vi "LIA Debugging Host.vi"() -> ()   [LabVIEW 2018]
uses:
  Shared/lib/host/Public/pll settings.ctl
  Shared/lib/host/Public/lock-in settings.ctl
  Class/LIA Debugging.lvclass
  C:/Users/jfernand/Repositories/Lock-In-Amplifier/Shared/lib/interface/Interface/LIA Host Interface.lvclass
  C:/Users/jfernand/Repositories/Lock-In-Amplifier/Shared/lib/interface/Interface FPGA/LIA Host Interface FPGA.lvclass
  <vilib>/Analysis/4window.llb/windowTd.ctl
  <vilib>/measure/maspectr.llb/FFT Power Spectrum and PSD for N Chan.vi
  <vilib>/Utility/error.llb/Error Cluster From Error Code.vi
  <vilib>/rvi/errors/niLvFpgaAdjustHostInterfaceError.vi
  <vilib>/rvi/interface/nirviReadWriteControl/nirviReadWriteControl.xnode
  Shared/lib/host/Lock-In Amplifier Example Host.lvlib
  <vilib>/Analysis/NI_AALPro.lvlib
  <vilib>/measure/NI_MAPro.lvlib
  <vilib>/Analysis/NI_AALBase.lvlib
  NiFpgaLv.dll
  <vilib>/rvi/interface/Simulation/niFpgaSimulationCallBeginRW.vi
  Shared/lib/interface/Interface FPGA/LIA Host Interface FPGA.lvclass
panel:
  in  "Tab Control 2":enum32{"Page 1", "Page 2"}(tab)
  in  "dpll.m 0":i8=-20
  in  "lock-in.decimator0 0":enum16{"None", "CIC", "FIR", "4HB", "SOS"}(ring)=enum."FIR"
  in  "lock-in.decimator1 0":enum16{"None", "FIR", "SOS"}(ring)=enum."FIR"
  in  "lock-in.iir config":T1={"b0"=0.001556396484375, "b1"=-0.000762939453125, "-a1"=1.9305267333984375, "-a2"=-0.9328765869140625} {"b0" format="%.17g"; "b1" format="%.17g"; "-a1" format="%.17g"; "-a2" format="%.17g"}
  out "lock-in.max-min":dbl=1.9775797561733533e-07 caption="Deviation" format="%#_6p"
  out "lock-in.min":dbl=1.9775797561733533e-07 caption="Deviation" format="%#_6p"
  out "lock-in.max":dbl=1.9775797561733533e-07 caption="Deviation" format="%#_6p"
  in  "Tab Control 1":T2(tab)
  out "pll.vco output 0":fxp<+/-,48,0> format="%#.18g"
  out "lock-in.cic config 0":cluster{"factor":fxp<+,16,16>, "shift":i16}
  out "dpll.vco output 0":fxp<+/-,48,0> format="%#.18g"
  out "dpll.config 0":T3
  out "nco.frequency 0":fxp<+/-,48,0>=0.0010000000000012221 format="%#_19g"
  out "stream.state 0":T4(ring)
  out "lock-in.decimator0 0 read":enum16{"None", "CIC", "FIR", "4HB", "SOS"}(ring)
  out "size(s)":i32
  out "lock-in.carrier 0 read":fxp<+/-,48,0> format="%_19g"
  out "stream.overflow? 0":bool
  out "Power Spectrum (dBm)":cluster{"f0":dbl, "df":dbl, "magnitude":dbl[]}(graph)
  out "Waveform Graph 3":dbl[][](graph)
  out "Waveform Graph 4":dbl[][](graph)
  out "Waveform Graph 6":waveform(dbl)[](graph)
  out "Waveform Graph":cluster{"f0":dbl, "df":dbl, "magnitude":dbl[]}[](graph)
  in  "app.quit":bool
  in  "lock-in.record length 0":u32=2048 caption="Record Length"
  in  "app.tab 0":enum32{"Lock-In", "PLL"}(tab)
  in  "lock-in.decimation1 0":i32=64 caption="Decimation 1"
  in  "lock-in.sampling rate":dbl=100000000.0 caption="Sampling Rate" format="%_10p"
  in  "lock-in.decimation0 0":i32=16 caption="Decimation 0"
  in  "lock-in.source 0":enum16{"AI 0", "AI 1", "AI 2", "AI 3", "NCO 0"}(ring)=enum."AI 1" caption="Channel"
  in  "lock-in.carrier 0":T5(ring)=enum."DPLL 0" caption="Carrier Source"
  in  "lock-in.manual carrier 0":dbl=100000.0 caption="Carrier Frequency" format="%_10p"
  in  "pll.source 0":enum16{"AI 0", "AI 1", "AI 2", "AI 3"}(ring) caption="Source"
  in  "pll.q frequency 0":dbl=100000.0 caption="Q Frequency" format="%#_6p"
  in  "pll.reset 0":bool caption="PLL Reset"
  in  "rio device":tag="PXI2Slot2" caption="Resource"
  out "lock-in.deviation":dbl=1.9775797561733533e-07 caption="Deviation" format="%#_6p"
  out "lock-in.mean":dbl=8.221341747482856e-05 format="%#_12p"
  out "Result":cluster{dbl, "standard deviation":dbl}(graph)
  # "NI Lock-In Amplifier Reference Example"
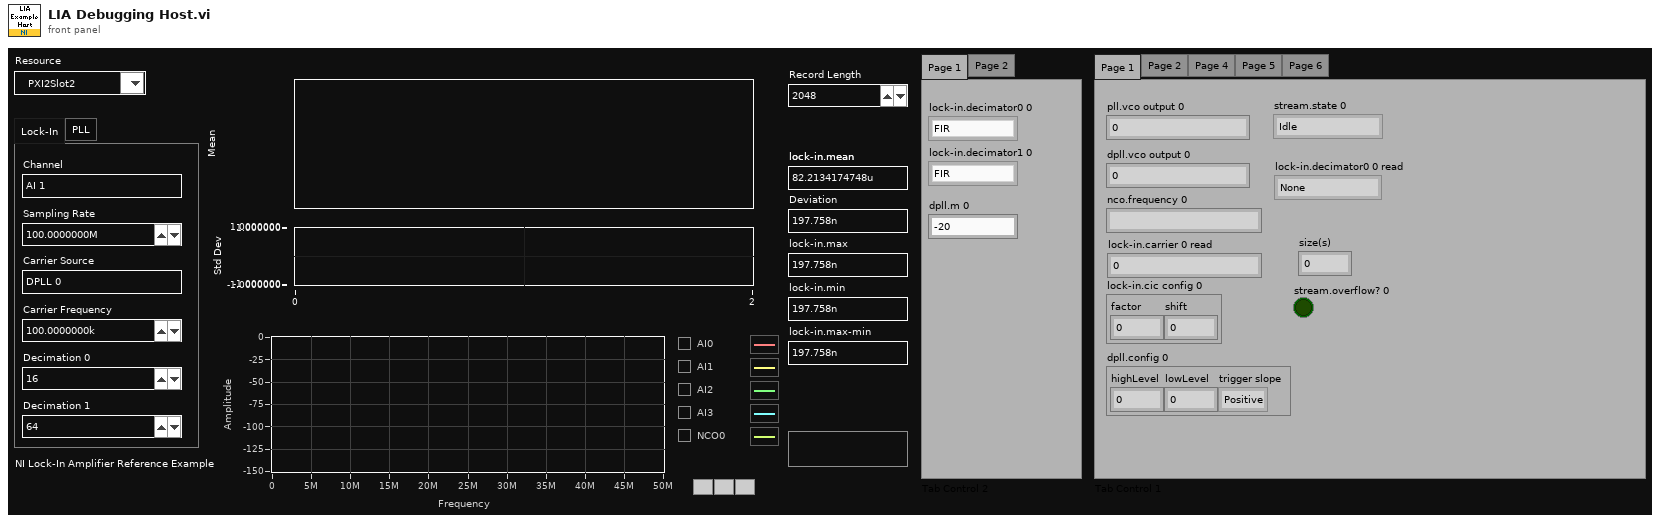
[diagram p1: front panel]
types:
  T1 = cluster{"b0":fxp<+/-,18,2>, "b1":fxp<+/-,18,2>, "-a1":fxp<+/-,18,2>, "-a2":fxp<+/-,18,2>}
  T2 = enum32{"Page 1", "Page 2", "Page 4", "Page 5", "Page 6"}
  T3 = cluster{"highLevel":fxp<+/-,18,1>, "lowLevel":fxp<+/-,18,1>, "trigger slope":enum8{"Positive", "Negative"}}
  T4 = enum8{"Idle", "Finite Transfer", "Continuous", "Done", "Error", "Not Ready", "Cancel"}
  T5 = enum16{"Manual 0", "Manual 1", "Manual 2", "Manual 3", "PLL 0", "PLL 1", "DPLL 0", "DPLL 1"}
  T6 = typedef "Lock-In Amplifier Example Host.lvlib/lock-in settings.ctl" = cluster{"decimation":i32, "source":i32, "carrier source":i32, "carrier":dbl}
  T7 = typedef "Lock-In Amplifier Example Host.lvlib/pll settings.ctl" = cluster{"source":i32, "q frequency":dbl}
  T8 = typedef "NI_AALPro.lvlib/windowTd.ctl" = u32
  T9 = enum16{"None", "CIC", "FIR", "4HB", "SOS", "4SOS"}
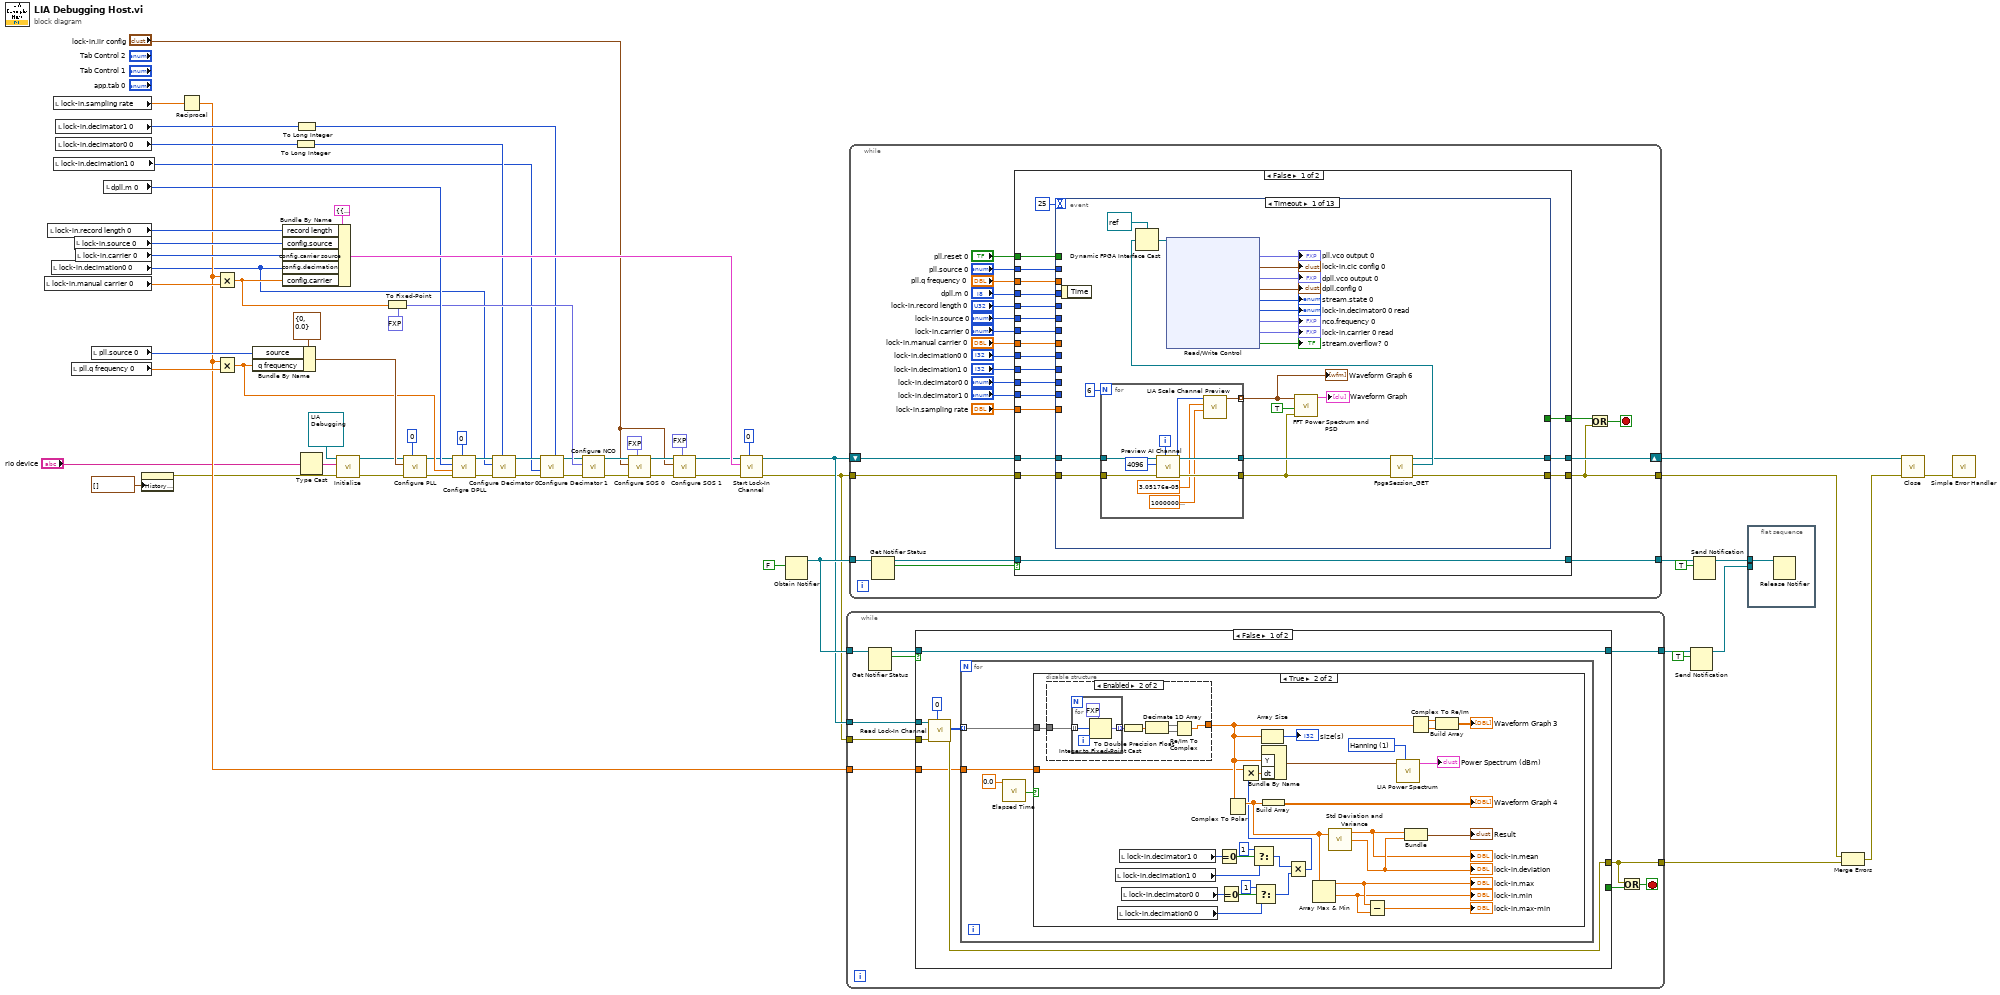
[diagram p0: block diagram]
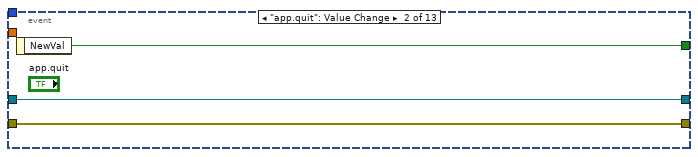
[diagram p2: hidden frame]
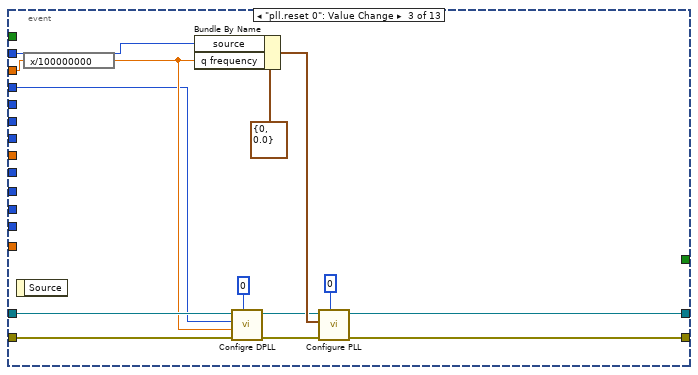
[diagram p3: hidden frame]
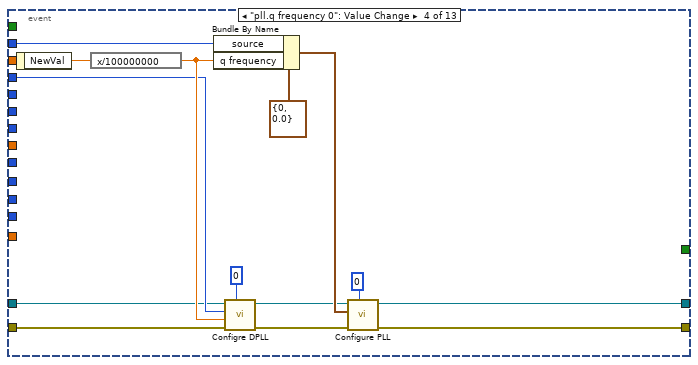
[diagram p4: hidden frame]
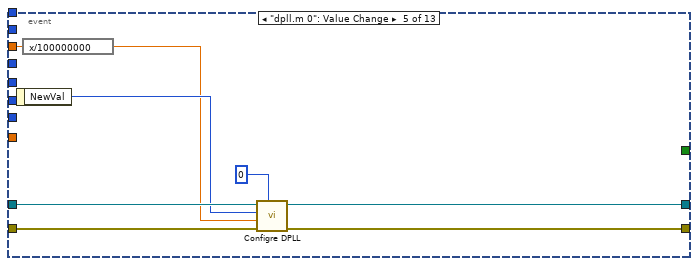
[diagram p5: hidden frame]
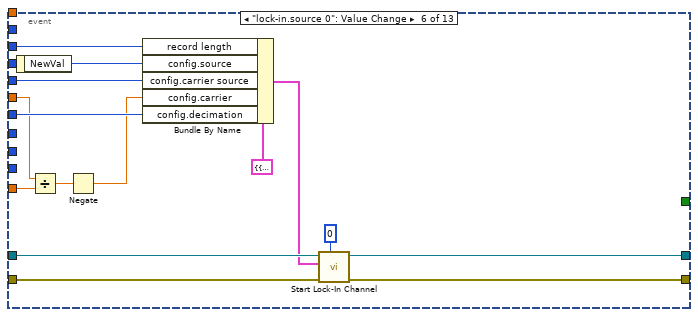
[diagram p6: hidden frame]
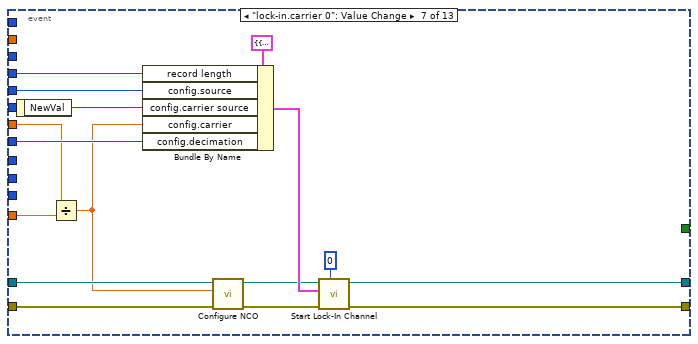
[diagram p7: hidden frame]
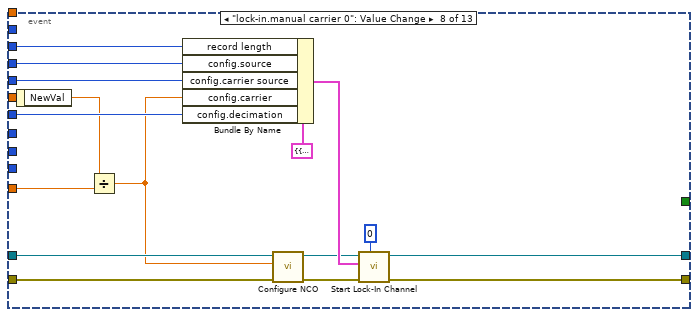
[diagram p8: hidden frame]
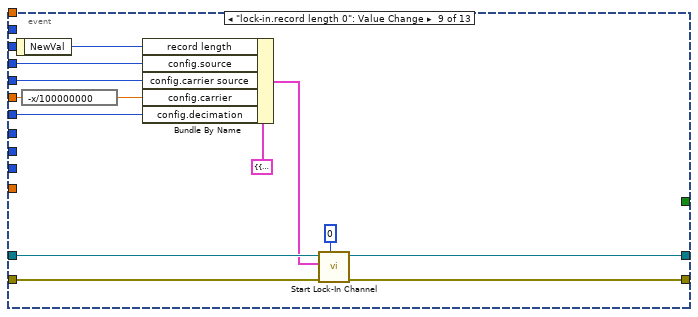
[diagram p9: hidden frame]
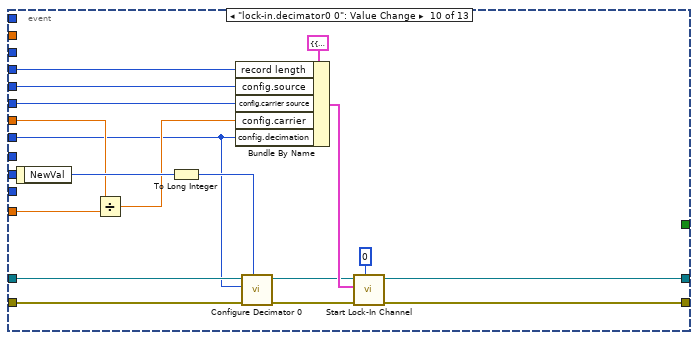
[diagram p10: hidden frame]
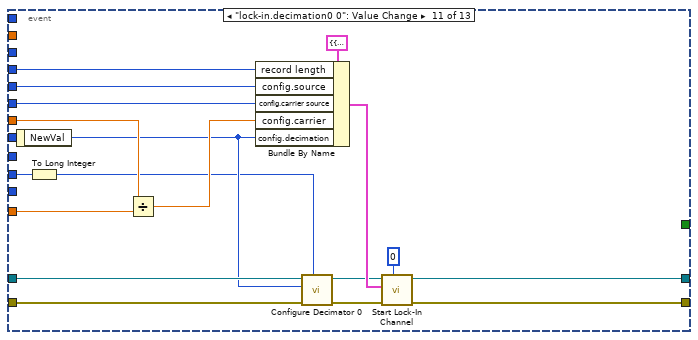
[diagram p11: hidden frame]
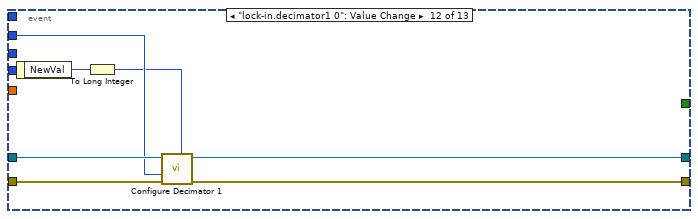
[diagram p12: hidden frame]
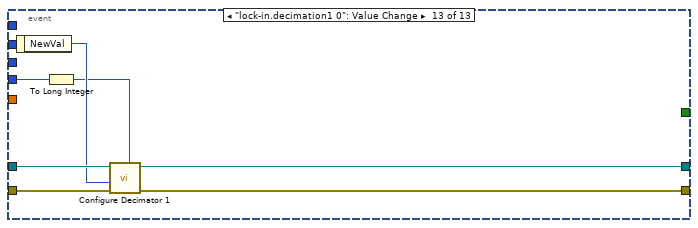
[diagram p13: hidden frame]
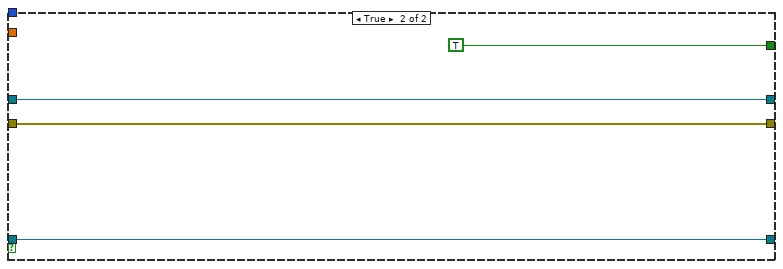
[diagram p14: hidden frame]
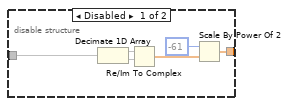
[diagram p16: hidden frame]
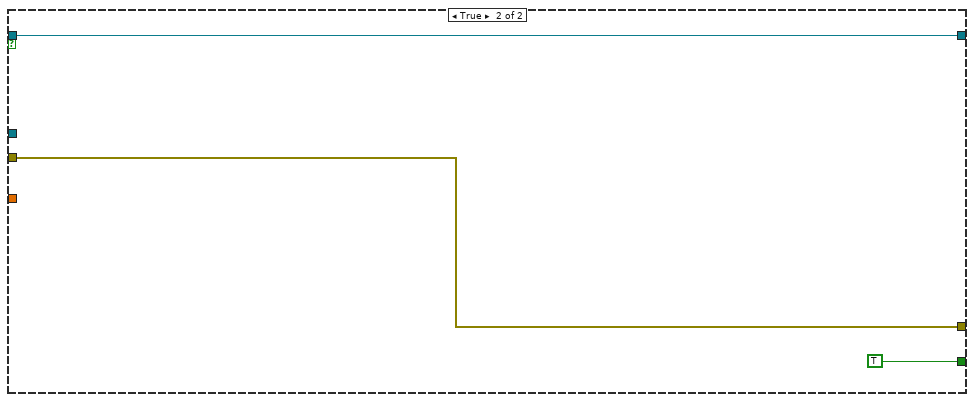
[diagram p17: hidden frame]
diagram:
  n1 = local read "lock-in.manual carrier 0"() -> (w60:dbl)
  n2 = local read "lock-in.record length 0"() -> (w43:u32)
  n3 = local read "lock-in.decimation0 0"() -> (w9:i32)
  n4 = local read "lock-in.sampling rate"() -> (w33:dbl)
  n5 = local read "lock-in.decimation1 0"() -> (w10:i32)
  n6 = local read "lock-in.decimator1 0"() -> (w29:enum16{"None", "FIR", "SOS"})
  n7 = local read "lock-in.decimator0 0"() -> (w28:enum16{"None", "CIC", "FIR", "4HB", "SOS"})
  n8 = local read "pll.q frequency 0"() -> (w61:dbl)
  n9 = local read "lock-in.source 0"() -> (w65:enum16{"AI 0", "AI 1", "AI 2", "AI 3", "NCO 0"})
  n10 = local read "lock-in.carrier 0"() -> (w64:T5)
  n11 = local read "pll.source 0"() -> (w62:enum16{"AI 0", "AI 1", "AI 2", "AI 3"})
  n12 = local read "dpll.m 0"() -> (w38:i8)
  n13 = property on="Result" class="WFChart (strict)"("History Data"=cluster{dbl, "standard deviation":dbl}[] []) -> (error out=w18:errorcluster)  [unwired: 2 in, 1 out]
  n14 = Reciprocal(x=w33) -> (1/x=w20:dbl)
  n15 = Multiply(x=w20, y=w60) -> (x*y=w21:dbl)
  n16 = Multiply(x=w20, y=w61) -> (x*y=w36:dbl)
  n17 = Bundle By Name(cluster=T7 {"source"=0, "q frequency"=0.0} ("config"), "source"=w62, "q frequency"=w36) -> (w37:T7)
  n18 = Bundle By Name(cluster=cluster{"config":T6, "record length":u32} {"config"={"decimation"=0, "source"=0, "carrier source"=0, "carrier"=0.0}, "record length"=0} ("config"), "record length"=w43, "config.source"=w65, "config.carrier source"=w64, "config.decimation"=w9, "config.carrier"=w21) -> (w44:cluster{"config":T6, "record length":u32})
  n19 = To Long Integer(number=w28) -> (32bit integer=w11:i32)
  n20 = To Long Integer(number=w29) -> (32bit integer=w12:i32)
  n21 = Type Cast(x="rio device") -> (*(type *) &x=w8:string)  [unwired: 1 in]
  n22 = call-dynamic "Initialize.vi"("error in"=w18, "resource"=w8, "host in"=refnum<class "LIA Debugging.lvclass"> refnum ("LIA Debugging.lvclass")) -> ("error out"=w22:errorcluster, "host out"=w23:refnum<class "LIA Debugging.lvclass">)  [unwired: 7 in]
  n23 = To Fixed-Point(fixed-point type=fxp<+/-,48,0> 0.0 ("nco.frequency 0"), number=w21) -> (fixed-point=w35:fxp<+/-,48,0>)
  n24 = call-dynamic "Configure PLL.vi"("index"=0, "error in"=w22, "config"=w37, "host in"=w23) -> ("error out"=w26:errorcluster, "host out"=w27:refnum<class "LIA Debugging.lvclass">)  [unwired: 6 in]
  n25 = call "Configre DPLL.vi"("dpll.channel 0"=0, "error in (no error)"=w26, "dpll.q 0"=w36, "dpll.m 0"=w38, "LIA Host Interface in"=w27) -> ("error out"=w39:errorcluster, "LIA Host Interface Out"=w40:refnum<class "LIA Debugging.lvclass">)  [unwired: 5 in]
  n26 = call-dynamic "Configure Decimator 0.vi"("lock-in.decimator0 0"=w11, "error in (no error)"=w39, "lock-in.decimation0 0"=w9, "LIA Host Interface in"=w40) -> ("error out"=w14:errorcluster, "LIA Host Interface out"=w16:refnum<class "LIA Debugging.lvclass">)  [unwired: 6 in]
  n27 = call "Configure Decimator 1.vi"("lock-in.decimator1 0"=w12, "error in (no error)"=w14, "lock-in.decimation1 0"=w10, "LIA Host Interface in"=w16) -> ("error out"=w13:errorcluster, "LIA Host Interface out"=w15:refnum<class "LIA Debugging.lvclass">)  [unwired: 6 in]
  n28 = call "Configure NCO.vi"("error in (no error)"=w13, "nco.frequency 0"=w35, "LIA Host Interface in"=w15) -> ("error out"=w30:errorcluster, "LIA Host Interface out"=w31:refnum<class "LIA Debugging.lvclass">)  [unwired: 7 in]
  n29 = call "Configure SOS 0.vi"("lock-in.iir decimation0 0"=fxp<+,4,4> 1.0, "error in (no error)"=w30, "lock-in.iir config 0 0"="lock-in.iir config", "LIA Host Interface in"=w31) -> ("error out"=w6:errorcluster, "LIA Host Interface out"=w7:refnum<class "LIA Debugging.lvclass">)  [unwired: 6 in]
  n30 = call "Configure SOS 1.vi"("lock-in.iir decimation1 0"=fxp<+,4,4> 1.0, "error in (no error)"=w6, "lock-in.iir config 1 0"="lock-in.iir config", "LIA Host Interface in"=w7) -> ("error out"=w4:errorcluster, "LIA Host Interface out"=w5:refnum<class "LIA Debugging.lvclass">)  [unwired: 6 in]
  n31 = call-dynamic "Start Lock-In Channel.vi"("index"=0, "error in"=w4, "config"=w44, "host in"=w5) -> ("error out"=w24:errorcluster, "host out"=w25:refnum<class "LIA Debugging.lvclass">)  [unwired: 6 in]
  n32 = Obtain Notifier(notification data type=FALSE) -> (notifier out=w57:refnum<notifier>)  [unwired: 3 in, 2 out]
  n33 = while {
    tunnel: w57 -> [w75]
    tunnel: w25 -> [w72]
    tunnel: w24 -> [w71]
    tunnel: [w70] -> w50
    tunnel: [w67] -> w53
    tunnel: w20 -> [w66]
    stop <- w69 stop-if-true
    n34 = Get Notifier Status(notifier=w75) -> (notifier out=w73:refnum<notifier>, current notification=w74:bool)  [unwired: 1 in, 3 out]
    n35 = case shown="False" w74 {
      tunnel: [w79 w134] -> w67
      tunnel: w73 -> [w79 w134]
      tunnel: w72 -> [w82 _]
      tunnel: w71 -> [w81 w133]
      tunnel: [w77 w133] -> w70
      tunnel: [_ TRUE] -> w68
      tunnel: w66 -> [w76 _]
      frame False {
        n36 = call-dynamic "Read Lock-In Channel.vi"("index"=0, "error in"=w81, "host in"=w82) -> ("error out"=w77:errorcluster, "unscaled data"=w78:i64[][])  [unwired: 6 in, 1 out]
        n37 = for {
          tunnel: w78 -> [w83] mode=indexing
          tunnel: w76 -> [w84]
          n38 = call "Elapsed Time"("Time Target (s)"=0.0) -> ("Time has Elapsed"=w86:bool)  [unwired: 11 in, 7 out]
          n39 = case shown="True" w86 {
            tunnel: w84 -> [_ w103]
            tunnel: w83 -> [_ w89]
            frame False {
            }
            frame True {
              w88 = T8 1 items=["Rectangle"=0, "Hanning"=1, "Hamming"=2, "Blackman-Harris"=3, "Exact Blackman"=4, "Blackman"=5, "Flat Top"=6, "4 Term B-Harris "=7, "7 Term B-Harris"=8, "Low Sidelobe"=9, "Blackman Nuttall"=11, "Triangle"=30, "Bartlett-Hanning"=31, "Bohman"=32, "Parzen"=33, "Welch"=34, "Kaiser"=60, "Dolph-Chebyshev"=61, "Gaussian"=62] ("window")
              n40 = disable-structure shown="Enabled" {
                disable-tunnel: [w121 w124] -> w105
                disable-tunnel: w89 -> [w117 w128]
                frame Disabled {
                  n41 = Decimate 1D Array(w117) -> (w120:i64[], w119:i64[])
                  n42 = Re/Im To Complex(1:w119, 2:w120) -> (0:w118:cdb[])
                  n43 = Scale By Power Of 2(n=i16 -61, x=w118) -> (x*2^n=w121:cdb[])
                }
                frame Enabled {
                  n44 = for {
                    tunnel: w128 -> [w131] mode=indexing
                    tunnel: [w129] -> w125 mode=indexing
                    n45 = Integer to Fixed-Point Cast(fixed-point type=fxp<+/-,64,1> 0.0, integer=w131) -> (fixed-point=w129:fxp<+/-,64,1>)
                  }
                  n46 = To Double Precision Float(number=w125) -> (double precision float=w123:dbl[])
                  n47 = Decimate 1D Array(w123) -> (w127:dbl[], w126:dbl[])
                  n48 = Re/Im To Complex(1:w126, 2:w127) -> (0:w124:cdb[])
                }
              }
              n49 = local read "lock-in.decimation1 0"() -> (w92:i32)
              n50 = local read "lock-in.decimation0 0"() -> (w100:i32)
              n51 = local read "lock-in.decimator1 0"() -> (w94:enum16{"None", "FIR", "SOS"})
              n52 = local read "lock-in.decimator0 0"() -> (w98:enum16{"None", "CIC", "FIR", "4HB", "SOS"})
              n53 = Equal To 0?(x=w94) -> (x = 0?=w93:bool)
              n54 = Equal To 0?(x=w98) -> (x = 0?=w99:bool)
              n55 = Complex To Polar(r * e^(i*theta)=w105) -> (r=w107:dbl[])  [unwired: 1 out]
              n56 = Select(t=1, s=w93, f=w92) -> (s? t:f=w91:i32)
              n57 = Select(t=1, s=w99, f=w100) -> (s? t:f=w96:i32)
              n58 = Array Size(array=w105) -> (size(s)=→"size(s)":i32)
              n59 = Build Array(w107) -> (→"Waveform Graph 4":dbl[][])
              n60 = Multiply(x=w91, y=w96) -> (x*y=w101:i32)
              n61 = Multiply(x=w103, y=w101) -> (x*y=w102:dbl)
              n62 = Bundle By Name("Y"=w105, "dt"=w102) -> (w87:waveform(cdb))  [unwired: 1 in]
              n63 = Array Max & Min(array=w107) -> (max value=w114:dbl, min value=w113:dbl)  [unwired: 2 out]
              "lock-in.max" <- w114
              "lock-in.min" <- w113
              n64 = call <vilib>:"Std Deviation and Variance.vi"("X"=w107) -> ("mean"=w106:dbl, "standard deviation"=w112:dbl)  [unwired: 1 in, 1 out]
              "lock-in.deviation" <- w112
              "lock-in.mean" <- w106
              n65 = Subtract(x=w114, y=w113) -> (x-y=→"lock-in.max-min":dbl)
              n66 = call "LIA Power Spectrum.vi"("window"=w88, "waveform"=w87) -> ("Waveform Graph 5"=→"Power Spectrum (dBm)":cluster{"x0":dbl, "dx":dbl, "Y":dbl[]})  [unwired: 9 in]
              n67 = Bundle("mean"=w106, "standard deviation"=w112) -> (→"Result":cluster{"mean":dbl, "standard deviation":dbl})  [unwired: 1 in]
              n68 = Complex To Re/Im(x + iy=w105) -> (x=w110:dbl[], y=w109:dbl[])
              n69 = Build Array(w110, w109) -> (→"Waveform Graph 3":dbl[][])
            }
          }
        }
      }
      frame True {
      }
    }
    n70 = Or(x=w70, y=w68) -> (x .or. y?=w69:bool)
  }
  n71 = while {
    tunnel: w24 -> [w157]
    shift-right: [w149] -> w59
    shift-left: w25 -> [w156]
    tunnel: [w145] -> w49
    tunnel: w57 -> [w148]
    tunnel: [w143] -> w56
    stop <- w155 stop-if-true
    n72 = Get Notifier Status(notifier=w148) -> (notifier out=w147:refnum<notifier>, current notification=w146:bool)  [unwired: 1 in, 3 out]
    n73 = case shown="False" w146 {
      tunnel: w157 -> [w177 w361]
      tunnel: w156 -> [w176 w362]
      tunnel: [w175 w361] -> w145
      tunnel: "lock-in.manual carrier 0" -> [w173 _]
      tunnel: "lock-in.decimation0 0" -> [w172 _]
      tunnel: "lock-in.source 0" -> [w171 _]
      tunnel: "lock-in.carrier 0" -> [w170 _]
      tunnel: "pll.source 0" -> [w169 _]
      tunnel: "pll.q frequency 0" -> [w168 _]
      tunnel: [w167 w362] -> w149
      tunnel: w147 -> [w165 w359]
      tunnel: [w166 TRUE] -> w144
      tunnel: [w165 w359] -> w143
      tunnel: "lock-in.record length 0" -> [w164 _]
      tunnel: "dpll.m 0" -> [w163 _]
      tunnel: "lock-in.decimator0 0" -> [w162 _]
      tunnel: "lock-in.sampling rate" -> [w161 _]
      tunnel: "pll.reset 0" -> [w160 _]
      tunnel: "lock-in.decimator1 0" -> [w159 _]
      tunnel: "lock-in.decimation1 0" -> [w158 _]
      frame False {
        n74 = event shown="[0] Timeout" {
          selector: _ -> [_ _ _ _ _ _ _ _ _ _ _ _ _]
          dyn-events: _ -> [_ _ _ _ _ _ _ _ _ _ _ _ _]
          timeout: 25 -> [_ _ _ _ _ _ _ _ _ _ _ _ _]
          tunnel: w177 -> [w198 w211 w216 w227 w243 w261 w269 w282 w304 w316 w334 w350 w355]
          tunnel: w176 -> [w199 w212 w218 w228 w248 w259 w271 w284 w302 w317 w335 w351 w356]
          tunnel: [w195 w211 w226 w236 w241 w260 w278 w293 w303 w315 w333 w345 w357] -> w175
          tunnel: w171 -> [_ _ _ _ _ _ w272 w287 w296 w323 w341 _ _]
          tunnel: w170 -> [_ _ _ _ _ w263 _ w295 w307 w326 w344 _ _]
          tunnel: w173 -> [_ _ _ _ w245 w251 w266 _ w306 w312 w331 _ _]
          tunnel: w172 -> [_ _ _ _ _ w262 w279 w294 w305 w309 _ _ _]
          tunnel: w169 -> [_ _ w223 w239 _ _ _ _ _ _ _ _ _]
          tunnel: w168 -> [_ _ w220 _ _ _ _ _ _ _ _ _ _]
          tunnel: [w181 w212 w221 w237 w242 w258 w264 w292 w301 w325 w343 w346 w358] -> w167
          tunnel: [_ w210 _ _ _ _ _ _ _ _ _ _ _] -> w166
          tunnel: w164 -> [_ _ _ _ _ w255 w275 w289 _ w321 w339 _ _]
          tunnel: w163 -> [_ _ w213 w231 _ _ _ _ _ _ _ _ _]
          tunnel: w162 -> [_ _ _ _ _ _ _ _ _ _ w330 _ _]
          tunnel: w161 -> [_ _ _ _ _ w250 w267 w285 _ w313 w332 _ _]
          tunnel: w160 -> [_ _ _ _ _ _ _ _ _ _ _ _ _]
          tunnel: w159 -> [_ _ _ _ _ _ _ _ _ _ _ _ w354]
          tunnel: w158 -> [_ _ _ _ _ _ _ _ _ _ _ w348 _]
          event Timeout {
            n75 = event-data() -> ()  [unwired: 1 in, 1 out]
            n76 = for {
              N: 6 -> [_]
              tunnel: w199 -> [w209]
              tunnel: [w207] -> w196
              tunnel: w198 -> [w208]
              tunnel: [w204] -> w187
              tunnel: [w202] -> w184 mode=indexing
              i -> [w205]
              n77 = call-dynamic "Preview AI Channel.vi"("index"=w205, "error in"=w208, "samples"=u32 4096, "host in"=w209) -> ("error out"=w204:errorcluster, "samples out"=w203:i16[], "host out"=w207:refnum<class "LIA Debugging.lvclass">)  [unwired: 5 in]
              n78 = call "LIA Scale Channel Preview.vi"("sample rate"=100000000.0, "scaling factor"=3.05176e-05, "ai data"=w203) -> ("Waveform"=w202:waveform(dbl))  [unwired: 8 in]
            }
            "Waveform Graph 6" <- w184
            n79 = call-poly <vilib>:"FFT Power Spectrum and PSD.vi"("error in (no error)"=w187, "dB On (F)"=TRUE, "time signals"=w184) -> ("Power Spectrum / PSD"=→"Waveform Graph":cluster{"f0":dbl, "df":dbl, "magnitude":dbl[]}[])  [unwired: 5 in, 3 out]
            n80 = call "FpgaSession_GET.vi"("error in"=w187, "lia host in"=w196) -> ("error out"=w195:errorcluster, "fpga session out"=w194:refnum<k20>, "lia host out"=w181:refnum<class "LIA Debugging.lvclass">)  [unwired: 7 in]
            n81 = Dynamic FPGA Interface Cast(Session In=refnum<k20> refnum ("fpga type"), Type=w194) -> (Session Out=w192:refnum<k20>)
            n82 = xnode "Read/Write Control"("FPGA VI Reference In"=w192) -> ("pll.vco output 0"=→"pll.vco output 0":fxp<+/-,48,0>, "lock-in.cic config 0"=→"lock-in.cic config 0":cluster{"factor":fxp<+,16,16>, "shift":i16}, "dpll.vco output 0"=→"dpll.vco output 0":fxp<+/-,48,0>, "dpll.config 0"=→"dpll.config 0":T3, "stream.state 0"=→"stream.state 0":T4, "lock-in.decimator0 0"=→"lock-in.decimator0 0 read":T9, "nco.frequency 0"=→"nco.frequency 0":fxp<+/-,48,0>, "lock-in.carrier 0"=→"lock-in.carrier 0 read":fxp<+/-,48,0>, "stream.overflow? 0"=→"stream.overflow? 0":bool)  [unwired: 1 in, 2 out]
          }
          event "app.quit": Value Change {
            n83 = event-data() -> ("NewVal"=w210:bool)  [unwired: 1 in]
          }
          event "pll.reset 0": Value Change {
            n84 = event-data() -> ()  [unwired: 1 in, 1 out]
            n85 = expression code="x/100000000"(w220) -> (w214:dbl)
            n86 = Bundle By Name(cluster=T7 {"source"=0, "q frequency"=0.0} ("config"), "source"=w223, "q frequency"=w214) -> (w222:T7)
            n87 = call "Configre DPLL.vi"("dpll.channel 0"=0, "error in (no error)"=w216, "dpll.q 0"=w214, "dpll.m 0"=w213, "LIA Host Interface in"=w218) -> ("error out"=w215:errorcluster, "LIA Host Interface Out"=w217:refnum<class "LIA Debugging.lvclass">)  [unwired: 5 in]
            n88 = call-dynamic "Configure PLL.vi"("index"=0, "error in"=w215, "config"=w222, "host in"=w217) -> ("error out"=w226:errorcluster, "host out"=w221:refnum<class "LIA Debugging.lvclass">)  [unwired: 6 in]
          }
          event "pll.q frequency 0": Value Change {
            n89 = event-data() -> ("NewVal"=w238:dbl)  [unwired: 1 in]
            n90 = expression code="x/100000000"(w238) -> (w232:dbl)
            n91 = Bundle By Name(cluster=T7 {"source"=0, "q frequency"=0.0} ("config"), "source"=w239, "q frequency"=w232) -> (w235:T7)
            n92 = call "Configre DPLL.vi"("dpll.channel 0"=0, "error in (no error)"=w227, "dpll.q 0"=w232, "dpll.m 0"=w231, "LIA Host Interface in"=w228) -> ("error out"=w229:errorcluster, "LIA Host Interface Out"=w230:refnum<class "LIA Debugging.lvclass">)  [unwired: 5 in]
            n93 = call-dynamic "Configure PLL.vi"("index"=0 ("instance"), "error in"=w229, "config"=w235, "host in"=w230) -> ("error out"=w236:errorcluster, "host out"=w237:refnum<class "LIA Debugging.lvclass">)  [unwired: 6 in]
          }
          event "dpll.m 0": Value Change {
            n94 = event-data() -> ("NewVal"=w246:i8)  [unwired: 1 in]
            n95 = expression code="x/100000000"(w245) -> (w244:dbl)
            n96 = call "Configre DPLL.vi"("dpll.channel 0"=0, "error in (no error)"=w243, "dpll.q 0"=w244, "dpll.m 0"=w246, "LIA Host Interface in"=w248) -> ("error out"=w241:errorcluster, "LIA Host Interface Out"=w242:refnum<class "LIA Debugging.lvclass">)  [unwired: 5 in]
          }
          event "lock-in.source 0": Value Change {
            n97 = event-data() -> ("NewVal"=w253:enum16{"AI 0", "AI 1", "AI 2", "AI 3", "NCO 0"})  [unwired: 1 in]
            n98 = Divide(x=w251, y=w250) -> (x/y=w252:dbl)
            n99 = Negate(x=w252) -> (-x=w249:dbl)
            n100 = Bundle By Name(cluster=cluster{"config":T6, "record length":u32} {"config"={"decimation"=0, "source"=0, "carrier source"=0, "carrier"=0.0}, "record length"=0} ("config"), "record length"=w255, "config.source"=w253, "config.carrier source"=w263, "config.carrier"=w249, "config.decimation"=w262) -> (w254:cluster{"config":T6, "record length":u32})
            n101 = call-dynamic "Start Lock-In Channel.vi"("index"=0, "error in"=w261, "config"=w254, "host in"=w259) -> ("error out"=w260:errorcluster, "host out"=w258:refnum<class "LIA Debugging.lvclass">)  [unwired: 6 in]
          }
          event "lock-in.carrier 0": Value Change {
            n102 = event-data() -> ("NewVal"=w273:T5)  [unwired: 1 in]
            n103 = Divide(x=w266, y=w267) -> (x/y=w265:dbl)
            n104 = Bundle By Name(cluster=cluster{"config":T6, "record length":u32} {"config"={"decimation"=0, "source"=0, "carrier source"=0, "carrier"=0.0}, "record length"=0} ("config"), "record length"=w275, "config.source"=w272, "config.carrier source"=w273, "config.carrier"=w265, "config.decimation"=w279) -> (w274:cluster{"config":T6, "record length":u32})
            n105 = call "Configure NCO.vi"("error in (no error)"=w269, "nco.frequency 0"=w265, "LIA Host Interface in"=w271) -> ("error out"=w268:errorcluster, "LIA Host Interface out"=w270:refnum<class "LIA Debugging.lvclass">)  [unwired: 7 in]
            n106 = call-dynamic "Start Lock-In Channel.vi"("index"=0, "error in"=w268, "config"=w274, "host in"=w270) -> ("error out"=w278:errorcluster, "host out"=w264:refnum<class "LIA Debugging.lvclass">)  [unwired: 6 in]
          }
          event "lock-in.manual carrier 0": Value Change {
            n107 = event-data() -> ("NewVal"=w286:dbl)  [unwired: 1 in]
            n108 = Divide(x=w286, y=w285) -> (x/y=w280:dbl)
            n109 = Bundle By Name(cluster=cluster{"config":T6, "record length":u32} {"config"={"decimation"=0, "source"=0, "carrier source"=0, "carrier"=0.0}, "record length"=0} ("config"), "record length"=w289, "config.source"=w287, "config.carrier source"=w295, "config.carrier"=w280, "config.decimation"=w294) -> (w288:cluster{"config":T6, "record length":u32})
            n110 = call "Configure NCO.vi"("error in (no error)"=w282, "nco.frequency 0"=w280, "LIA Host Interface in"=w284) -> ("error out"=w281:errorcluster, "LIA Host Interface out"=w283:refnum<class "LIA Debugging.lvclass">)  [unwired: 7 in]
            n111 = call-dynamic "Start Lock-In Channel.vi"("index"=0, "error in"=w281, "config"=w288, "host in"=w283) -> ("error out"=w293:errorcluster, "host out"=w292:refnum<class "LIA Debugging.lvclass">)  [unwired: 6 in]
          }
          event "lock-in.record length 0": Value Change {
            n112 = event-data() -> ("NewVal"=w297:u32)  [unwired: 1 in]
            n113 = expression code="-x/100000000"(w306) -> (w308:dbl)
            n114 = Bundle By Name(cluster=cluster{"config":T6, "record length":u32} {"config"={"decimation"=0, "source"=0, "carrier source"=0, "carrier"=0.0}, "record length"=0} ("config"), "record length"=w297, "config.source"=w296, "config.carrier source"=w307, "config.carrier"=w308, "config.decimation"=w305) -> (w298:cluster{"config":T6, "record length":u32})
            n115 = call-dynamic "Start Lock-In Channel.vi"("index"=0, "error in"=w304, "config"=w298, "host in"=w302) -> ("error out"=w303:errorcluster, "host out"=w301:refnum<class "LIA Debugging.lvclass">)  [unwired: 6 in]
          }
          event "lock-in.decimator0 0": Value Change {
            n116 = event-data() -> ("NewVal"=w314:enum16{"None", "CIC", "FIR", "4HB", "SOS"})  [unwired: 1 in]
            n117 = Divide(x=w312, y=w313) -> (x/y=w311:dbl)
            n118 = To Long Integer(number=w314) -> (32bit integer=w310:i32)
            n119 = Bundle By Name(cluster=cluster{"config":T6, "record length":u32} {"config"={"decimation"=0, "source"=0, "carrier source"=0, "carrier"=0.0}, "record length"=0} ("config"), "record length"=w321, "config.source"=w323, "config.carrier source"=w326, "config.carrier"=w311, "config.decimation"=w309) -> (w320:cluster{"config":T6, "record length":u32})
            n120 = call-dynamic "Configure Decimator 0.vi"("lock-in.decimator0 0"=w310, "error in (no error)"=w316, "lock-in.decimation0 0"=w309, "LIA Host Interface in"=w317) -> ("error out"=w318:errorcluster, "LIA Host Interface out"=w319:refnum<class "LIA Debugging.lvclass">)  [unwired: 6 in]
            n121 = call-dynamic "Start Lock-In Channel.vi"("index"=0, "error in"=w318, "config"=w320, "host in"=w319) -> ("error out"=w315:errorcluster, "host out"=w325:refnum<class "LIA Debugging.lvclass">)  [unwired: 6 in]
          }
          event "lock-in.decimation0 0": Value Change {
            n122 = event-data() -> ("NewVal"=w328:i32)  [unwired: 1 in]
            n123 = To Long Integer(number=w330) -> (32bit integer=w327:i32)
            n124 = Divide(x=w331, y=w332) -> (x/y=w329:dbl)
            n125 = Bundle By Name(cluster=cluster{"config":T6, "record length":u32} {"config"={"decimation"=0, "source"=0, "carrier source"=0, "carrier"=0.0}, "record length"=0} ("config"), "record length"=w339, "config.source"=w341, "config.carrier source"=w344, "config.carrier"=w329, "config.decimation"=w328) -> (w338:cluster{"config":T6, "record length":u32})
            n126 = call-dynamic "Configure Decimator 0.vi"("lock-in.decimator0 0"=w327, "error in (no error)"=w334, "lock-in.decimation0 0"=w328, "LIA Host Interface in"=w335) -> ("error out"=w336:errorcluster, "LIA Host Interface out"=w337:refnum<class "LIA Debugging.lvclass">)  [unwired: 6 in]
            n127 = call-dynamic "Start Lock-In Channel.vi"("index"=0, "error in"=w336, "config"=w338, "host in"=w337) -> ("error out"=w333:errorcluster, "host out"=w343:refnum<class "LIA Debugging.lvclass">)  [unwired: 6 in]
          }
          event "lock-in.decimator1 0": Value Change {
            n128 = event-data() -> ("NewVal"=w349:enum16{"None", "FIR", "SOS"})  [unwired: 1 in]
            n129 = To Long Integer(number=w349) -> (32bit integer=w347:i32)
            n130 = call "Configure Decimator 1.vi"("lock-in.decimator1 0"=w347, "error in (no error)"=w350, "lock-in.decimation1 0"=w348, "LIA Host Interface in"=w351) -> ("error out"=w345:errorcluster, "LIA Host Interface out"=w346:refnum<class "LIA Debugging.lvclass">)  [unwired: 6 in]
          }
          event "lock-in.decimation1 0": Value Change {
            n131 = event-data() -> ("NewVal"=w353:i32)  [unwired: 1 in]
            n132 = To Long Integer(number=w354) -> (32bit integer=w352:i32)
            n133 = call "Configure Decimator 1.vi"("lock-in.decimator1 0"=w352, "error in (no error)"=w355, "lock-in.decimation1 0"=w353, "LIA Host Interface in"=w356) -> ("error out"=w357:errorcluster, "LIA Host Interface out"=w358:refnum<class "LIA Debugging.lvclass">)  [unwired: 6 in]
          }
        }
      }
      frame True {
      }
    }
    n134 = Or(x=w144, y=w145) -> (x .or. y?=w155:bool)
  }
  n135 = Send Notification(notification=TRUE, notifier=w53) -> (notifier out=w51:refnum<notifier>)  [unwired: 1 in, 1 out]
  n136 = Send Notification(notification=TRUE, notifier=w56) -> (notifier out=w52:refnum<notifier>)  [unwired: 1 in, 1 out]
  n137 = flat-sequence {
    tunnel: w52 -> [w363]
    tunnel: w51 -> [_]
    frame #0 {
      n138 = Release Notifier(notifier=w363) -> ()  [unwired: 2 in, 3 out]
    }
  }
  n139 = Merge Errors(w49, w50) -> (w48:errorcluster)
  n140 = call-dynamic "Close.vi"("error in"=w48, "host in"=w59) -> ("error out"=w42:errorcluster)  [unwired: 8 in, 1 out]
  n141 = call <vilib>:"Simple Error Handler.vi"("error in (no error)"=w42) -> ()  [unwired: 4 in, 5 out]
